vi "Edit_Raw_DF.vi"(5 "Edit Raw Data Header Info":bool, 7 "New Values In":string[](array[string])=[""], 8 "New Chs In":string[](array[string])=[""], 9 "Data filename":path) -> (0 "Filetype":string, 1 "Original values":string[](array[string]), 3 "Data filename out":path, 4 "File Not Changed?":bool)   [LabVIEW 2015]
uses:
  Globals/Constants_global.vi
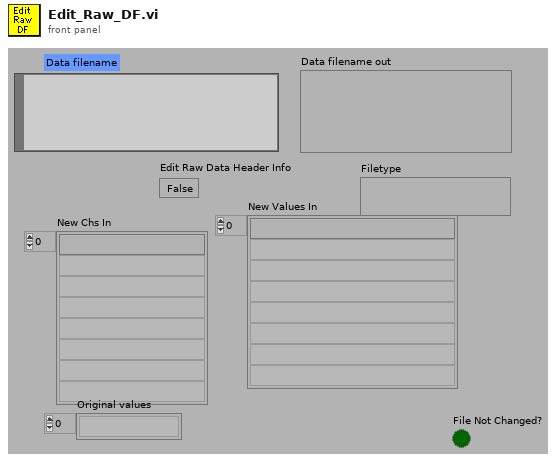
[diagram p1: front panel]
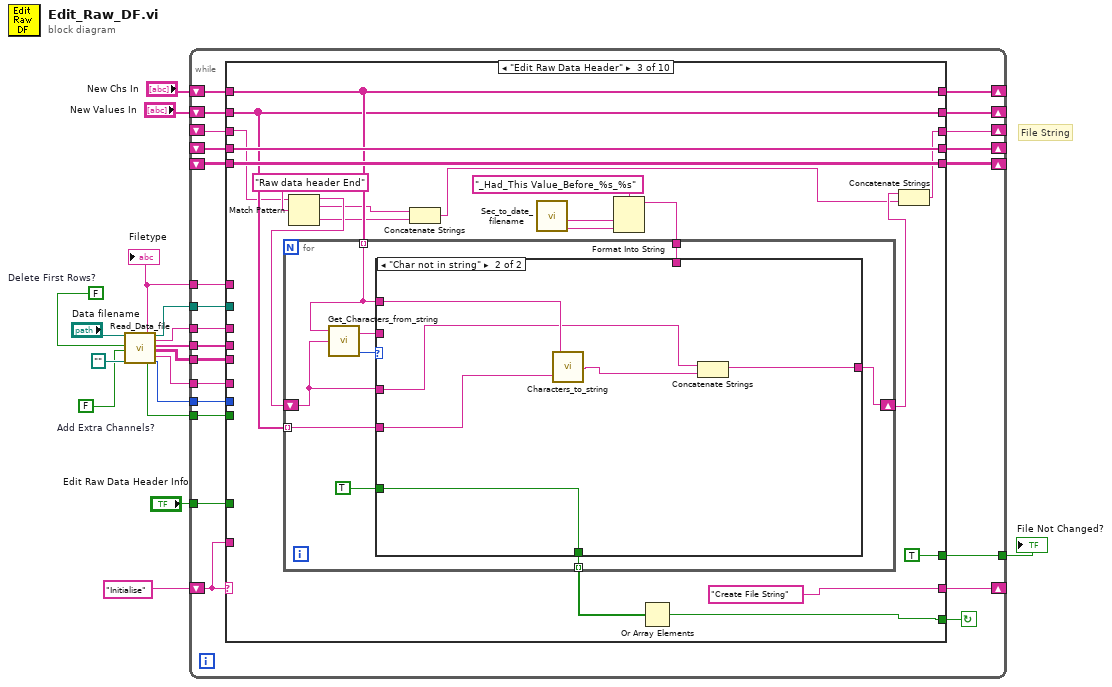
[diagram p0: block diagram]
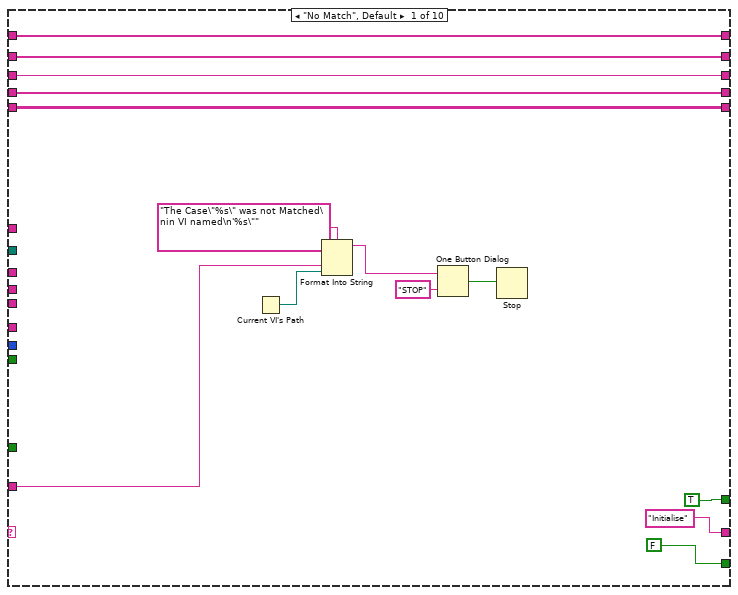
[diagram p2: hidden frame]
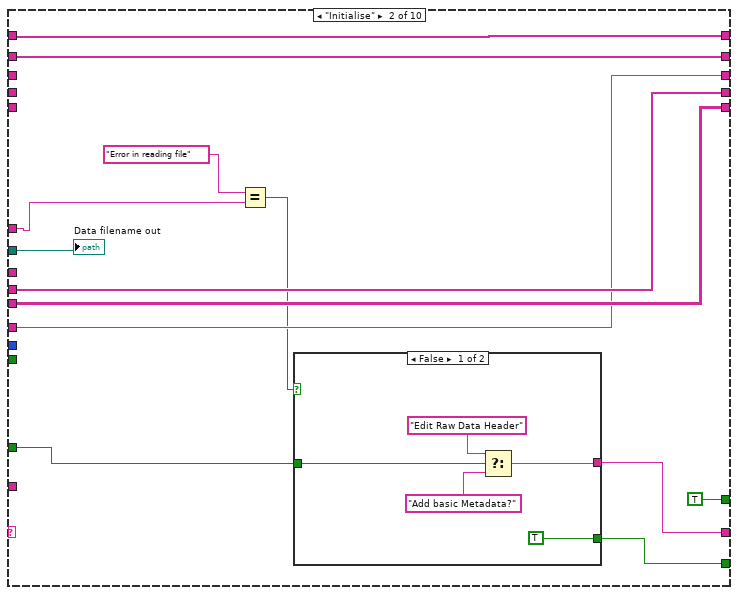
[diagram p3: hidden frame]
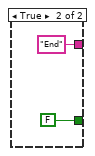
[diagram p4: hidden frame]
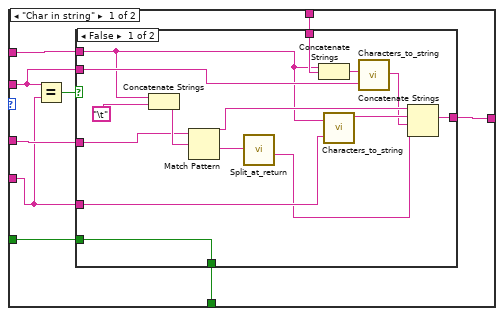
[diagram p5: hidden frame]
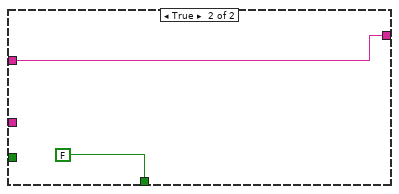
[diagram p6: hidden frame]
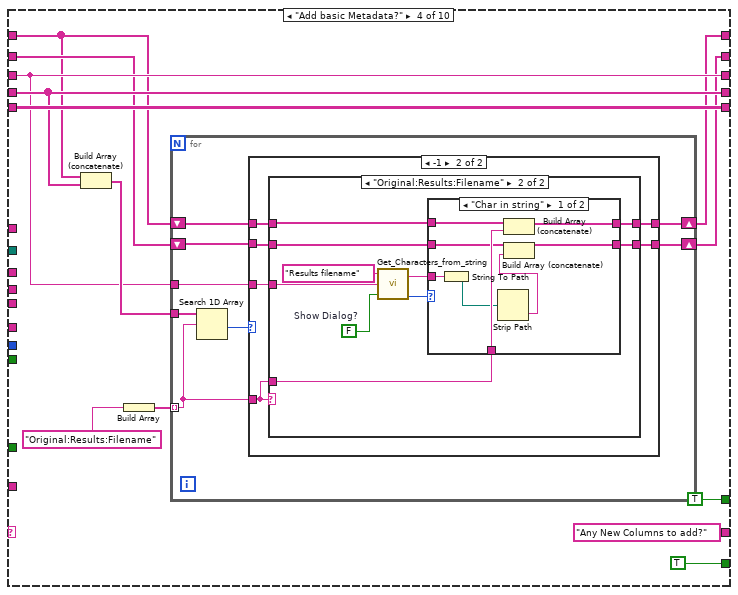
[diagram p7: hidden frame]
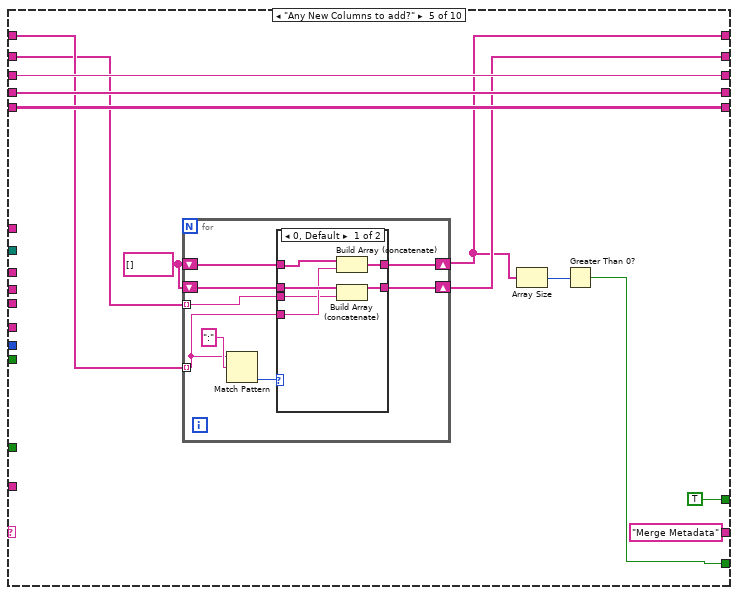
[diagram p11: hidden frame]
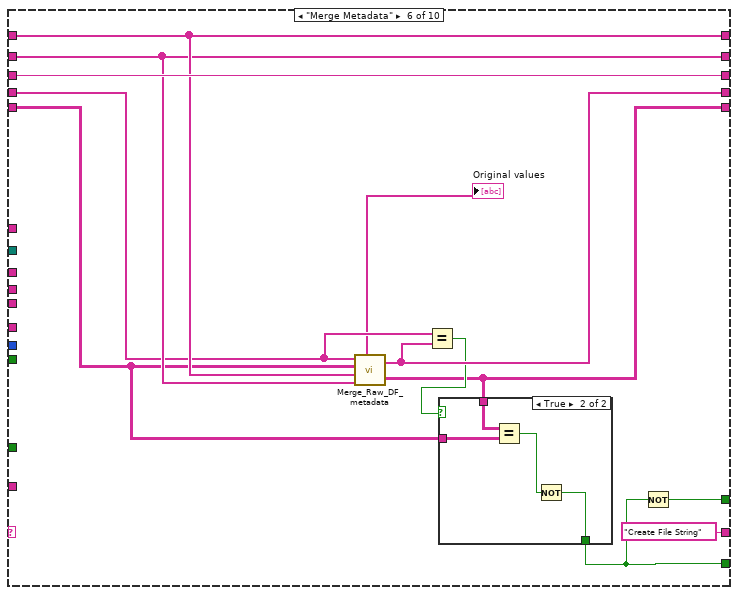
[diagram p13: hidden frame]
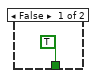
[diagram p14: hidden frame]
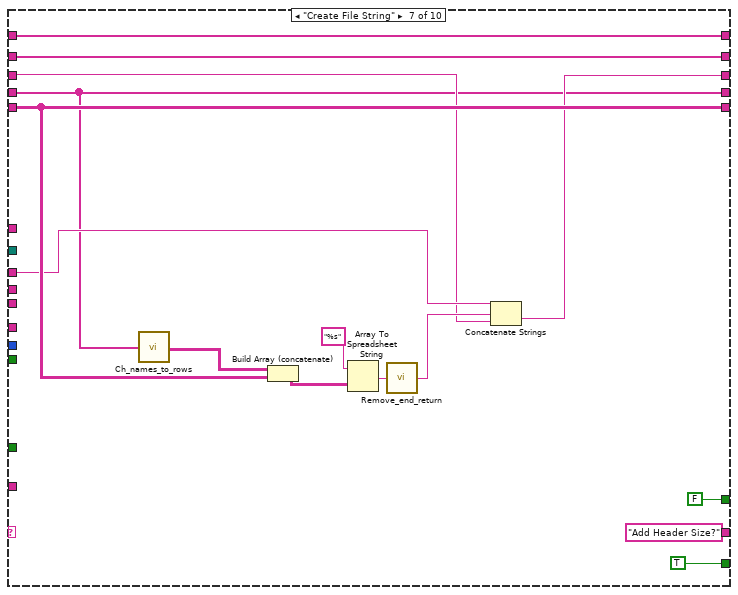
[diagram p15: hidden frame]
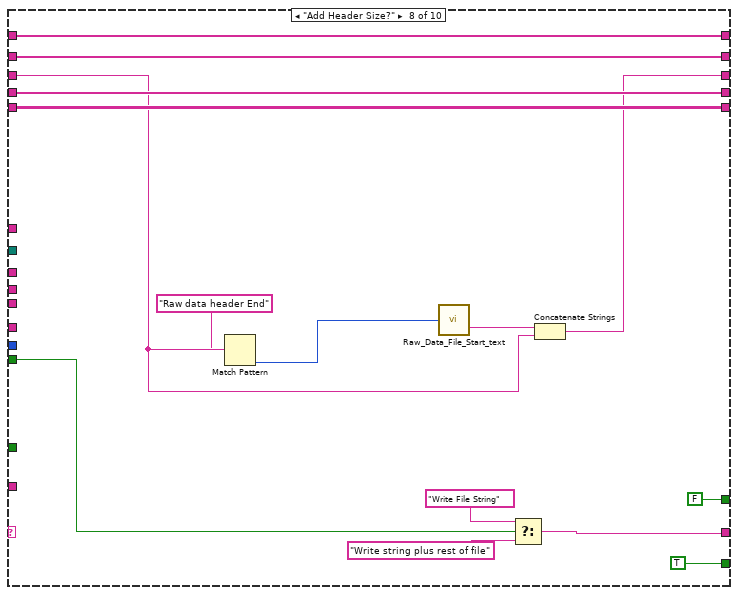
[diagram p16: hidden frame]
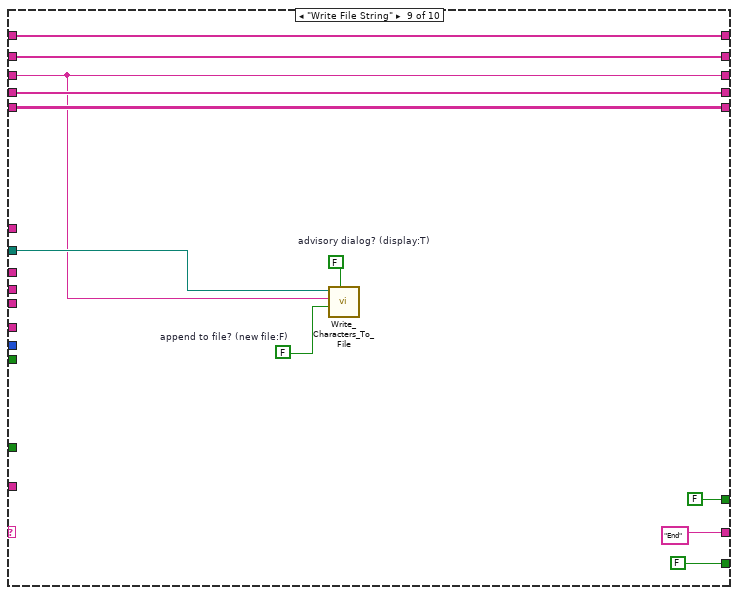
[diagram p17: hidden frame]
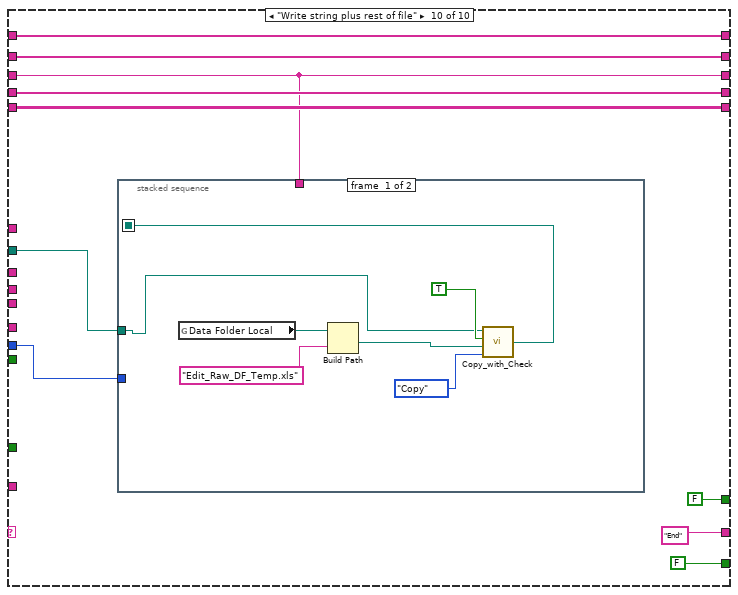
[diagram p18: hidden frame]
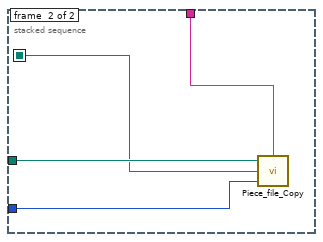
[diagram p19: hidden frame]
diagram:
  w1 = FALSE  # Delete First Rows?
  w15 = FALSE  # Add Extra Channels?
  # "File String"
  n1 = call "Read_Data_file.vi"("Results file"="Data filename", "Delete First Rows?"=w1, "Add Extra Channels?"=w15, "Template File"=path "") -> ("Filetype"=w10:string, "EOF?"=w8:bool, "Results file Out"=w13:path, "String Before"=w9:string, "Ch names Out"=w12:string[], "Channel Values Out"=w11:string[][], "String After"=w7:string, "mark after read (chars.)"=w6:i32)  [unwired: 2 in, 6 out]
  "Filetype" <- w10
  n2 = while {
    tunnel: "Edit Raw Data Header Info" -> [w19]
    shift-left: "New Values In" -> [w21]
    shift-right: [w20] -> _
    shift-left: "New Chs In" -> [w23]
    shift-right: [w22] -> _
    tunnel: w6 -> [w24]
    tunnel: w7 -> [w25]
    tunnel: w8 -> [w26]
    tunnel: w9 -> [w27]
    tunnel: w10 -> [w28]
    tunnel: w11 -> [w29]
    tunnel: w12 -> [w30]
    tunnel: w13 -> [w31]
    shift-left: _ -> [w32]
    shift-right: [w36] -> _
    shift-left: _ -> [w33]
    shift-right: [w35] -> _
    shift-left: _ -> [w34]
    shift-right: [w37] -> _
    shift-left: "Initialise" -> [w38]
    shift-right: [w39] -> _
    tunnel: [w18] -> w2
    stop <- w40 continue-if-true
    n3 = case shown="\"Edit Raw Data Header\"" w38 {
      tunnel: [FALSE w55 w76 TRUE w194 w217 TRUE TRUE FALSE FALSE] -> w40
      tunnel: ["Initialise" w59 "Create File String" ("f") "Any New Columns to add?" "Merge Metadata" ("f") "Create File String" ("f") "Add Header Size?" ("f") w255 "End" "End"] -> w39
      tunnel: w38 -> [w49 _ _ _ _ _ _ _ _ _]
      tunnel: [w46 w62 w79 w141 w198 w226 w239 w253 w267 w277] -> w37
      tunnel: [w44 w63 w94 w147 w197 w220 w241 w259 w270 w280] -> w36
      tunnel: [w45 w64 w93 w144 w196 w223 w233 w260 w271 w281] -> w35
      tunnel: w34 -> [w46 _ w85 w141 w198 w226 w235 w254 w267 w277]
      tunnel: w33 -> [w45 _ w93 w144 w196 w222 w233 w260 w271 w281]
      tunnel: w32 -> [w44 _ w94 w147 w197 w219 w241 w259 w270 w280]
      tunnel: w31 -> [_ w67 _ _ _ _ _ _ w268 w278]
      tunnel: w30 -> [_ w64 _ _ _ _ _ _ _ _]
      tunnel: w29 -> [_ w63 _ _ _ _ _ _ _ _]
      tunnel: w28 -> [_ w57 _ _ _ _ _ _ _ _]
      tunnel: w27 -> [_ _ _ _ _ _ w240 _ _ _]
      tunnel: w26 -> [_ _ _ _ _ _ _ w256 _ _]
      tunnel: w25 -> [_ w62 _ _ _ _ _ _ _ _]
      tunnel: w24 -> [_ _ _ _ _ _ _ _ _ w276]
      tunnel: w23 -> [w43 w66 w88 w137 w190 w225 w237 w252 w264 w275]
      tunnel: [w43 w66 w88 w140 w188 w225 w237 w252 w264 w275] -> w22
      tunnel: w21 -> [w42 w65 w87 w138 w189 w224 w236 w251 w263 w274]
      tunnel: [w42 w65 w87 w139 w191 w224 w236 w251 w263 w274] -> w20
      tunnel: w19 -> [_ w60 _ _ _ _ _ _ _ _]
      tunnel: [TRUE TRUE TRUE TRUE TRUE w216 FALSE FALSE FALSE FALSE] -> w18
      frame "No Match", Default {
        n4 = Current VI's Path() -> (path=w48:path)
        n5 = Format Into String(format string="The Case\"%s\" was not Matched\nin VI named\n'%s\"" ("Format String"), w49, w48) -> (resulting string=w52:string)  [unwired: 2 in, 1 out]
        n6 = One Button Dialog(message=w52, button name ("OK")="STOP") -> (true=w50:bool)
        n7 = Stop(stop? (T)=w50) -> ()
      }
      frame "Initialise" {
        n8 = Equal?(x="Error in reading file", y=w57) -> (x = y?=w56:bool)
        n9 = case shown="False" w56 {
          tunnel: w60 -> [w70 _]
          tunnel: [w69 "End"] -> w59
          tunnel: [TRUE FALSE] -> w55
          frame False {
            n10 = Select(t="Edit Raw Data Header", s=w70, f="Add basic Metadata?") -> (s? t:f=w69:string)
          }
          frame True {
          }
        }
        "Data filename out" <- w67
      }
      frame "Edit Raw Data Header" {
        n11 = Match Pattern(string=w85, regular expression="Raw data header End") -> (before substring=w84:string, match substring=w83:string, after substring=w82:string)  [unwired: 2 out]
        n12 = Concatenate Strings(w83, w82) -> (w80:string)
        n13 = call "Sec_to_date_filename.vi"() -> ("Day"=w90:string, "Time"=w75:string)  [unwired: 1 in, 2 out]
        n14 = Format Into String(format string="_Had_This Value_Before_%s_%s" ("Format String"), w90, w75) -> (resulting string=w91:string)  [unwired: 2 in, 1 out]
        n15 = for {
          shift-right: [w98] -> w81
          shift-left: w84 -> [w100]
          tunnel: w88 -> [w101] mode=indexing
          tunnel: w87 -> [w99] mode=indexing
          tunnel: w91 -> [w97]
          tunnel: [w96] -> w77 mode=indexing
          n16 = call "Get_Characters_from_string.vi"("Input string"=w100, "Variable name"=w101) -> ("Status"=w103:enum16{"Char in string", "Char not in string"}, "Value"=w102:string)  [unwired: 1 in]
          n17 = case shown="\"Char not in string\"" w103 {
            tunnel: w101 -> [w110 w135]
            tunnel: w99 -> [w109 w134]
            tunnel: [w111 w133] -> w98
            tunnel: w100 -> [w112 w132]
            tunnel: w102 -> [w107 _]
            tunnel: w97 -> [w106 _]
            tunnel: [w105 w130] -> w96
            tunnel: TRUE -> [w104 w130]
            frame "Char in string" {
              n18 = Equal?(x=w107, y=w109) -> (x = y?=w108:bool)
              n19 = case shown="False" w108 {
                tunnel: w112 -> [w125 w129]
                tunnel: [w123 w129] -> w111
                tunnel: w109 -> [w122 _]
                tunnel: w110 -> [w116 _]
                tunnel: w107 -> [w118 _]
                tunnel: w106 -> [w117 _]
                tunnel: [w113 FALSE] -> w105
                tunnel: w104 -> [w113 _]
                frame False {
                  n20 = Concatenate Strings(w116, "\t") -> (w126:string)
                  n21 = Match Pattern(string=w125, regular expression=w126) -> (before substring=w120:string, after substring=w124:string)  [unwired: 3 out]
                  n22 = call "Split_at_return.vi"("String"=w124) -> ("after substring"=w119:string)  [unwired: 1 in, 3 out]
                  n23 = Concatenate Strings(w116, w117) -> (w115:string)
                  n24 = call "Characters_to_string.vi"("Characters to write"=w122, "Label for characters"=w116) -> ("Output string"=w121:string)
                  n25 = call "Characters_to_string.vi"("Characters to write"=w118, "Label for characters"=w115) -> ("Output string"=w114:string)
                  n26 = Concatenate Strings(w120, w121, w114, w119) -> (w123:string)
                }
                frame True {
                }
              }
            }
            frame "Char not in string" {
              n27 = call "Characters_to_string.vi"("Characters to write"=w134, "Label for characters"=w135) -> ("Output string"=w131:string)
              n28 = Concatenate Strings(w132, w131) -> (w133:string)
            }
          }
        }
        n29 = Or Array Elements(Boolean array=w77) -> (logical OR=w76:bool)
        n30 = Concatenate Strings(w81, w80) -> (w79:string)
      }
      frame "Add basic Metadata?" {
        n31 = Build Array (concatenate)(w137, w144) -> (w142:string[])
        n32 = Build Array("Original:Results:Filename") -> (w143:string[])
        n33 = for {
          tunnel: w143 -> [w154] mode=indexing
          tunnel: w142 -> [w155]
          shift-right: [w153] -> w140
          shift-left: w137 -> [w152]
          shift-right: [w150] -> w139
          shift-left: w138 -> [w151]
          tunnel: w141 -> [w149]
          n34 = Search 1D Array(1D array=w155, element=w154) -> (index of element=w156:i32)  [unwired: 1 out]
          n35 = case shown="-1" w156 {
            tunnel: w154 -> [_ w159]
            tunnel: [w158 w164] -> w153
            tunnel: w152 -> [w158 w163]
            tunnel: w151 -> [w157 w162]
            tunnel: [w157 w161] -> w150
            tunnel: w149 -> [_ w160]
            frame 0, Default {
            }
            frame -1 {
              n36 = case shown="\"Original:Results:Filename\"" w159 {
                tunnel: [w166 w170] -> w164
                tunnel: w163 -> [w166 w172]
                tunnel: w162 -> [w165 w168]
                tunnel: [w165 w167] -> w161
                tunnel: w160 -> [_ w175]
                tunnel: w159 -> [_ w171]
                frame "Other", Default {
                }
                frame "Original:Results:Filename" {
                  w174 = FALSE  # Show Dialog?
                  n37 = call "Get_Characters_from_string.vi"("Show Dialog?"=w174, "Input string"=w175, "Variable name"="Results filename") -> ("Status"=w173:enum16{"Char in string", "Char not in string"}, "Value"=w169:string)
                  n38 = case shown="\"Char in string\"" w173 {
                    tunnel: w172 -> [w184 w186]
                    tunnel: w171 -> [w183 _]
                    tunnel: [w182 w186] -> w170
                    tunnel: w169 -> [w181 _]
                    tunnel: w168 -> [w179 w185]
                    tunnel: [w178 w185] -> w167
                    frame "Char in string" {
                      n39 = String To Path(string=w181) -> (path=w180:path)
                      n40 = Strip Path(path=w180) -> (name=w177:string)  [unwired: 1 out]
                      n41 = Build Array (concatenate)(w184, w183) -> (w182:string[])
                      n42 = Build Array (concatenate)(w179, w177) -> (w178:string[])
                    }
                    frame "Char not in string" {
                    }
                  }
                }
              }
            }
          }
        }
      }
      frame "Any New Columns to add?" {
        w192 = string[] []
        n43 = for {
          tunnel: w190 -> [w200] mode=indexing
          shift-right: [w201] -> w188
          shift-left: w192 -> [w204]
          shift-right: [w203] -> w191
          shift-left: w192 -> [w202]
          tunnel: w189 -> [w199] mode=indexing
          n44 = Match Pattern(string=w200, regular expression=":") -> (offset past match=w205:i32)  [unwired: 4 out]
          n45 = case shown="0, Default" w205 {
            tunnel: [w209 w214] -> w201
            tunnel: w204 -> [w212 w214]
            tunnel: [w210 w213] -> w203
            tunnel: w202 -> [w211 w213]
            tunnel: w200 -> [w208 _]
            tunnel: w199 -> [w207 _]
            frame 0, Default {
              n46 = Build Array (concatenate)(w212, w208) -> (w209:string[])
              n47 = Build Array (concatenate)(w211, w207) -> (w210:string[])
            }
            frame -1 {
            }
          }
        }
        n48 = Array Size(array=w188) -> (size(s)=w195:i32)
        n49 = Greater Than 0?(x=w195) -> (x > 0?=w194:bool)
      }
      frame "Merge Metadata" {
        n50 = call "Merge_Raw_DF_metadata.vi"("New Values In"=w224, "New Chs In"=w225, "Orig Values In"=w219, "Orig Chs In"=w222) -> ("Channel Values Out"=w220:string[][], "Ch names Out"=w223:string[], "Original values"=→"Original values":string[])  [unwired: 1 in]
        n51 = Equal?(x=w222, y=w223) -> (x = y?=w221:bool)
        n52 = case shown="True" w221 {
          tunnel: [TRUE w228] -> w217
          tunnel: w220 -> [_ w231]
          tunnel: w219 -> [_ w230]
          frame False {
          }
          frame True {
            n53 = Equal?(x=w231, y=w230) -> (x = y?=w229:bool)
            n54 = Not(x=w229) -> (.not. x?=w228:bool)
          }
        }
        n55 = Not(x=w217) -> (.not. x?=w216:bool)
      }
      frame "Create File String" {
        n56 = call "Ch_names_to_rows.vi"("Channel Names"=w233) -> ("3 Row names"=w232:string[][])
        n57 = Build Array (concatenate)(w232, w241) -> (w242:string[][])
        n58 = Array To Spreadsheet String(array=w242, 3:"%s" ("format string")) -> (spreadsheet string=w244:string)  [unwired: 1 out]
        n59 = call "Remove_end_return.vi"("Input string"=w244) -> ("Output string"=w245:string)
        n60 = Concatenate Strings(w240, w245, w235) -> (w239:string)
      }
      frame "Add Header Size?" {
        n61 = Match Pattern(string=w254, regular expression="Raw data header End") -> (offset past match=w248:i32)  [unwired: 4 out]
        n62 = call "Raw_Data_File_Start_text.vi"("Header length"=w248) -> ("Start String"=w247:string)
        n63 = Select(t="Write File String", s=w256, f="Write string plus rest of file") -> (s? t:f=w255:string)
        n64 = Concatenate Strings(w247, w254) -> (w253:string)
      }
      frame "Write File String" {
        w266 = FALSE  # append to file? (new file:F)
        w269 = FALSE  # advisory dialog? (display:T)
        n65 = call "Write_Characters_To_File.vi"("file path (dialog if empty)"=w268, "advisory dialog? (display:T)"=w269, "character string"=w267, "append to file? (new file:F)"=w266) -> ()  [unwired: 1 in, 4 out]
      }
      frame "Write string plus rest of file" {
        n66 = stacked-sequence {
          seq-local: [w283 _] -> [_ w291]
          tunnel: w278 -> [w284 w292]
          tunnel: w277 -> [_ w293]
          tunnel: w276 -> [_ w290]
          frame #0 {
            n67 = global read "Constants_global.vi" "Data Folder Local"() -> (w288:path)
            n68 = Build Path(base path=w288, name or relative path="Edit_Raw_DF_Temp.xls") -> (appended path=w285:path)
            n69 = call "Copy_with_Check.vi"("Mode"=enum16{"Move", "Copy"}."Copy", "Target Path"=w285, "Variable Target?"=TRUE, "Source Path"=w284) -> ("Pathname Out"=w283:path)
          }
          frame #1 {
            n70 = call "Piece_file_Copy.vi"("File Start String"=w293, "Start to copy file at:"=w290, "Source File"=w291, "Target File"=w292) -> ()  [unwired: 1 out]
          }
        }
      }
    }
  }
  "File Not Changed?" <- w2
